vi "ParseLines.vi"(8 "error in":errorcluster, 11 "Lines":string[](array[string])) -> (0 "error out":errorcluster, 3 "Config":T1)   [LabVIEW 2020]
uses:
  <vilib>/WebServerConfig/Config.ctl
  <vilib>/WebServerConfig/Server.ctl
  <vilib>/WebServerConfig/Alias.ctl
  <vilib>/WebServerConfig/ErrorDocument.ctl
  <vilib>/WebServerConfig/Action.ctl
  <vilib>/WebServerConfig/Redirect.ctl
  <vilib>/WebServerConfig/Interface.ctl
  <vilib>/WebServerConfig/AddHandler.ctl
  <vilib>/WebServerConfig/SSL.ctl
  <vilib>/WebServerConfig/CustomLog.ctl
  <vilib>/WebServerConfig/LoadModule.ctl
  <vilib>/regexp/Match Regular Expression.xnode
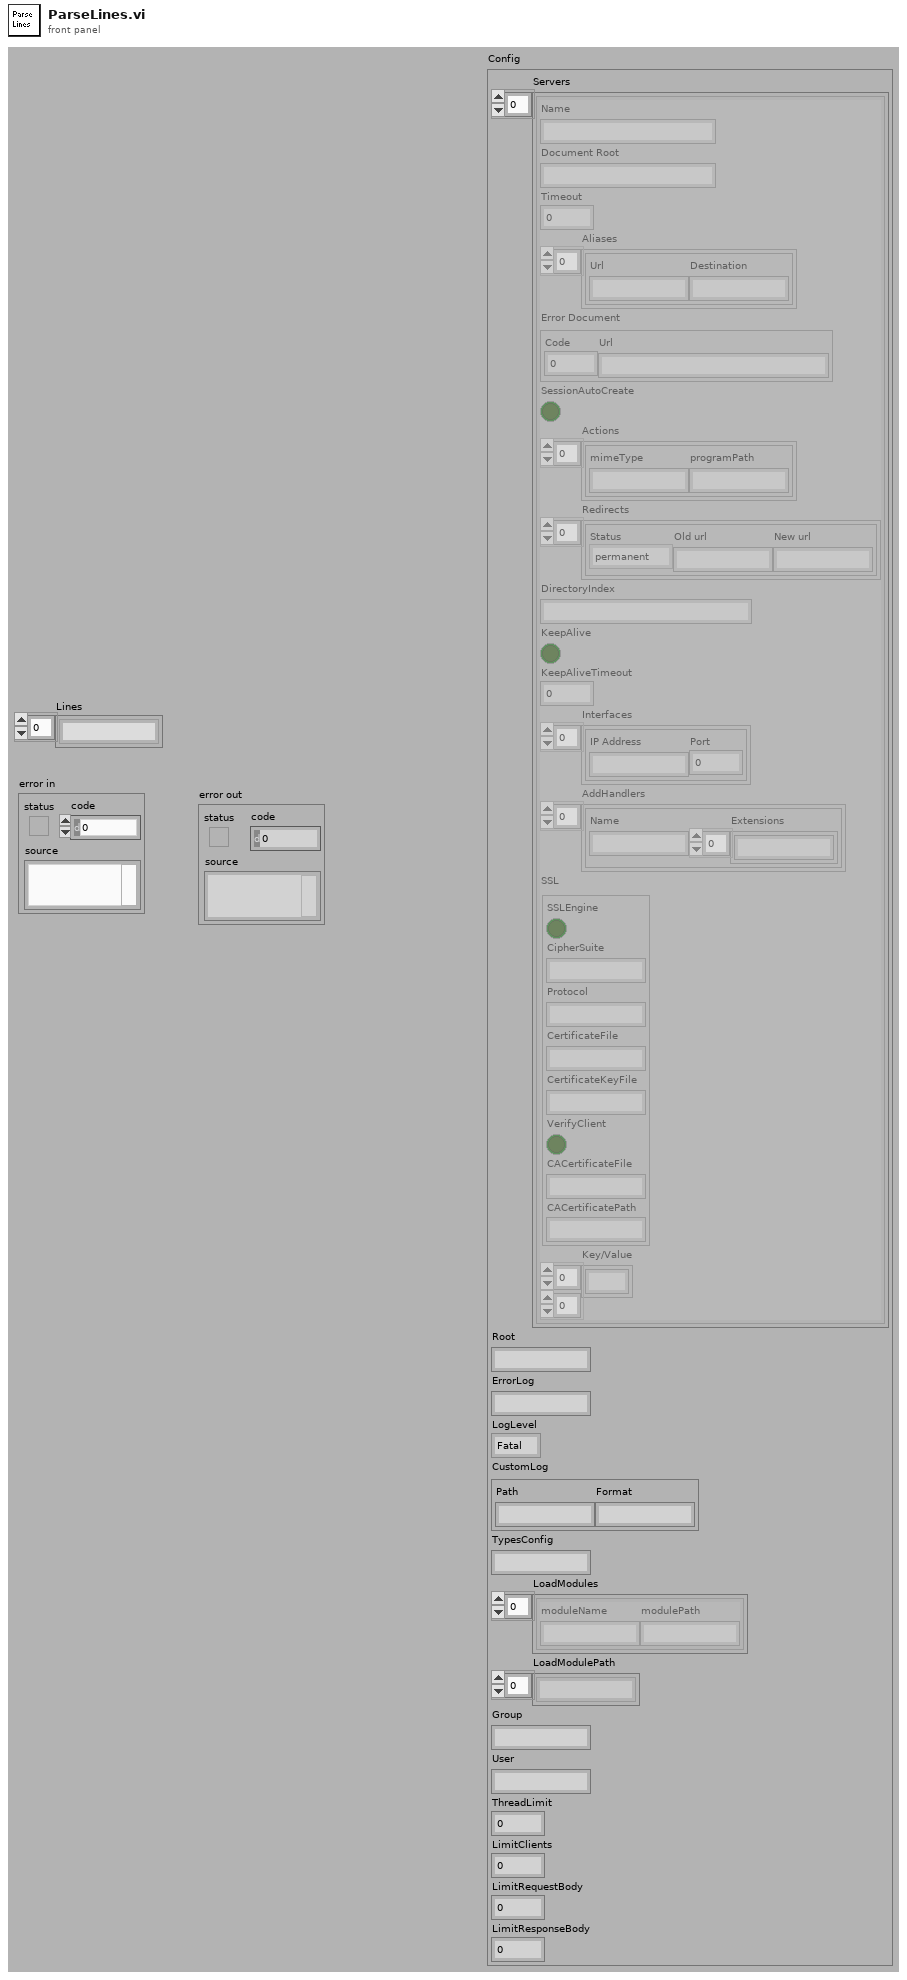
[diagram p1: front panel]
types:
  T1 = typedef "Config.ctl" = cluster{"Servers":T2[], "Root":string, "ErrorLog":string, "LogLevel":enum16{"Fatal", "Error", "Warn", "Info", "Debug", "5", "6", "7", "8", "Verbose"}, "CustomLog":T10, "TypesConfig":string, "LoadModules":T11[], "LoadModulePath":string[], "Group":string, "User":string, "ThreadLimit":u32, "LimitClients":u32, "LimitRequestBody":u32, "LimitResponseBody":u32}
  T2 = typedef "Server.ctl" = cluster{"Name":string, "Document Root":string, "Timeout":u32, "Aliases":T3[], "Error Document":T4, "SessionAutoCreate":bool, "Actions":T5[], "Redirects":T6[], "DirectoryIndex":string, "KeepAlive":bool, "KeepAliveTimeout":u32, "Interfaces":T7[], "AddHandlers":T8[], "SSL":T9, "Key/Value":string[][]}
  T3 = typedef "Alias.ctl" = cluster{"Url":string, "Destination":string}
  T4 = typedef "ErrorDocument.ctl" = cluster{"Code":u16, "Url":string}
  T5 = typedef "Action.ctl" = cluster{"mimeType":string, "programPath":string}
  T6 = typedef "Redirect.ctl" = cluster{"Status":enum16{"permanent", "temp", "seeother", "gone"}, "Old url":string, "New url":string}
  T7 = typedef "Interface.ctl" = cluster{"IP Address":string, "Port":u16}
  T8 = typedef "AddHandler.ctl" = cluster{"Name":string, "Extensions":string[]}
  T9 = typedef "SSL.ctl" = cluster{"SSLEngine":bool, "CipherSuite":string, "Protocol":string, "CertificateFile":string, "CertificateKeyFile":string, "VerifyClient":bool, "CACertificateFile":string, "CACertificatePath":string}
  T10 = typedef "CustomLog.ctl" = cluster{"Path":string, "Format":string}
  T11 = typedef "LoadModule.ctl" = cluster{"moduleName":string, "modulePath":string}
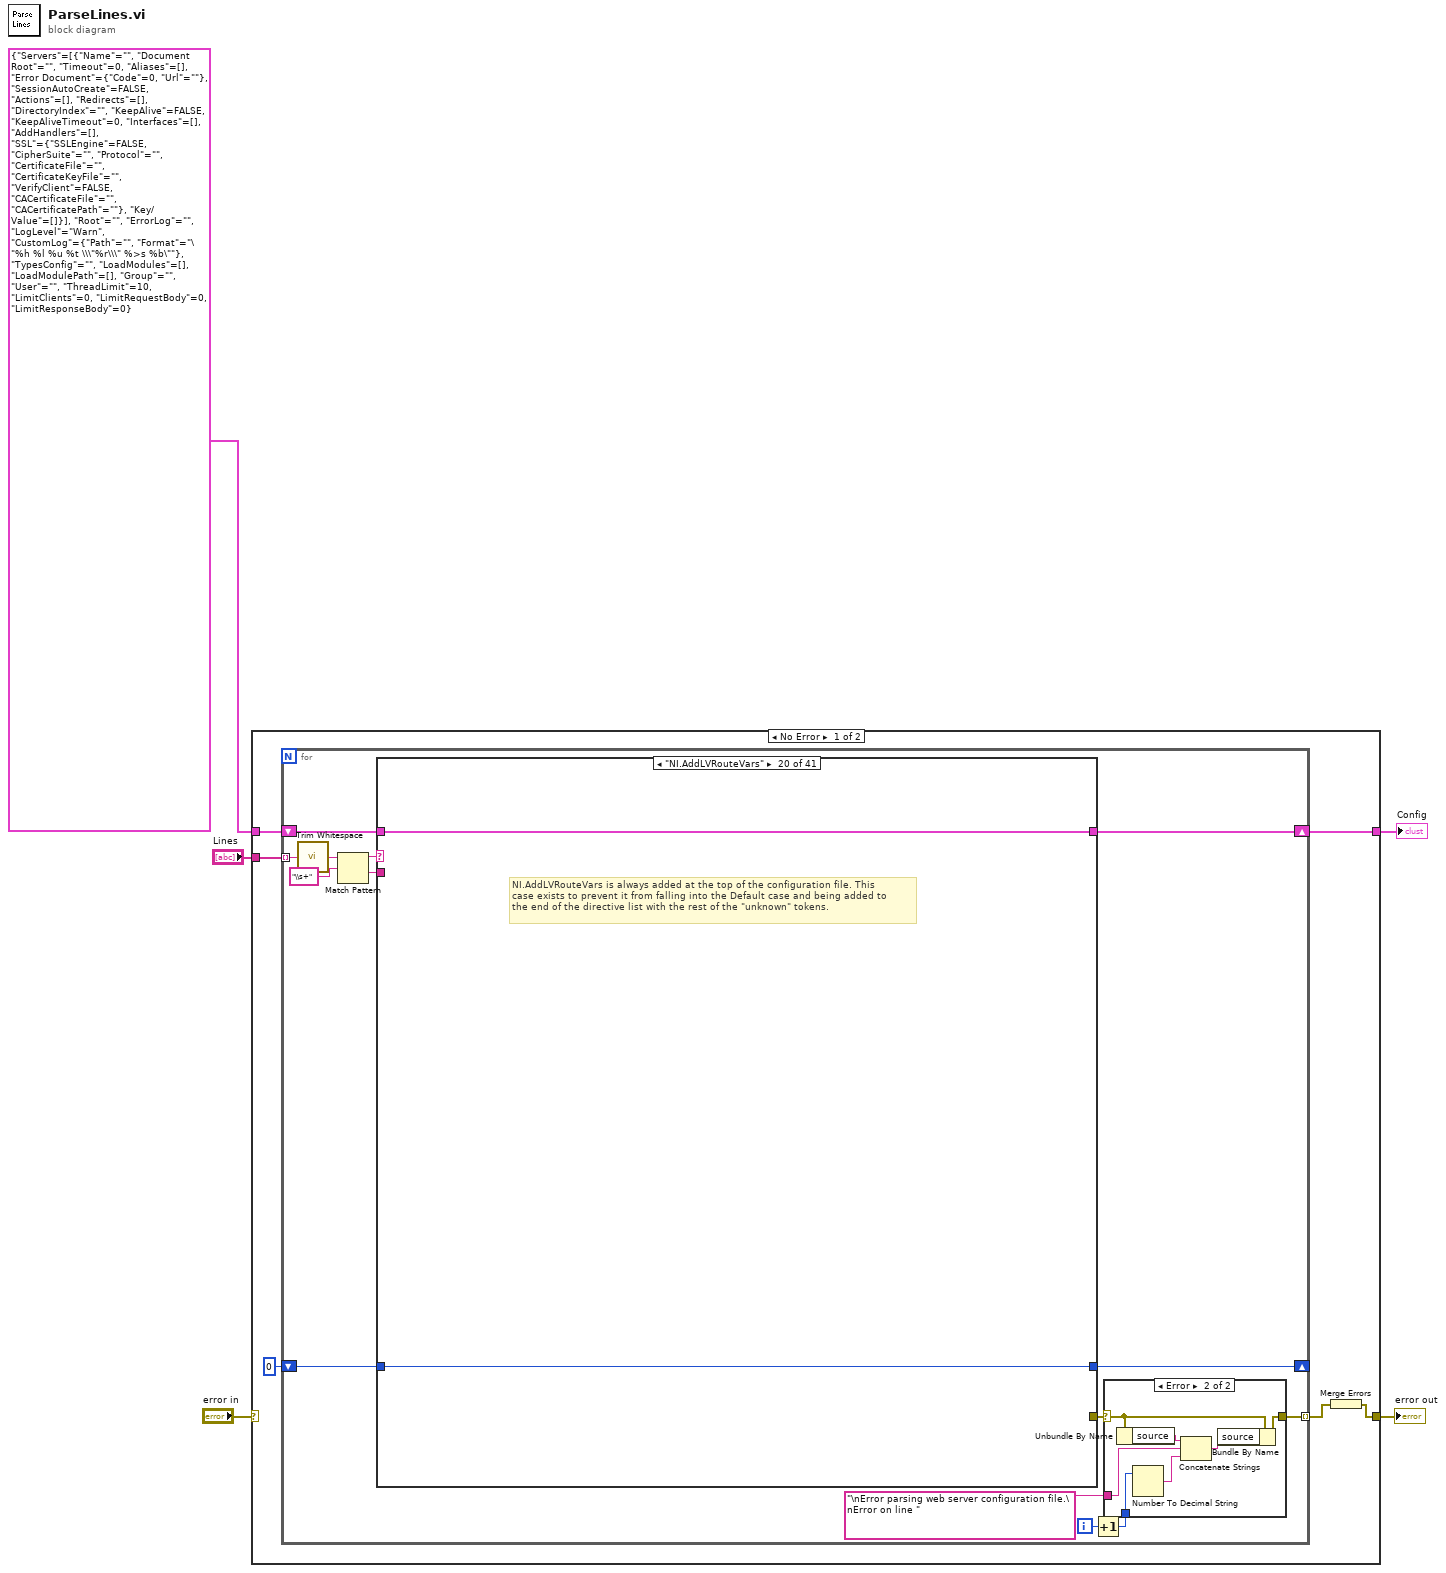
[diagram p0: block diagram]
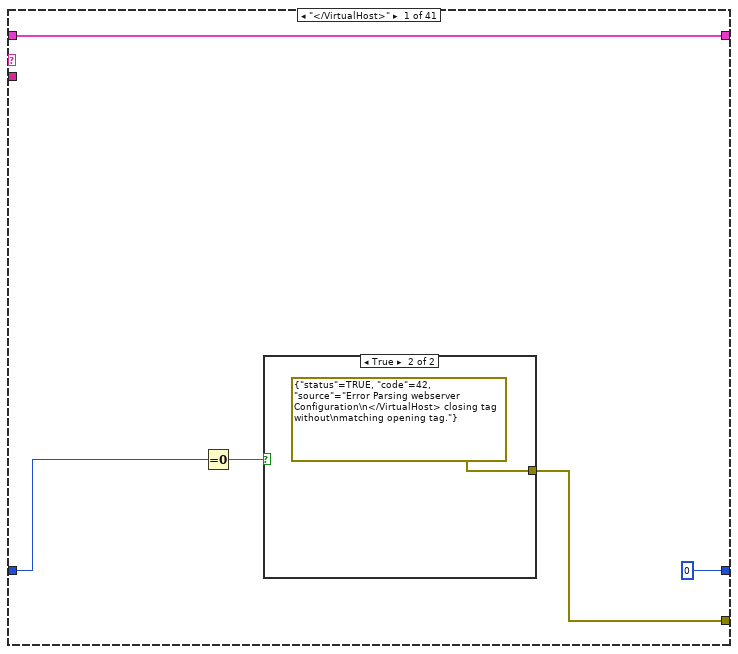
[diagram p3: hidden frame]
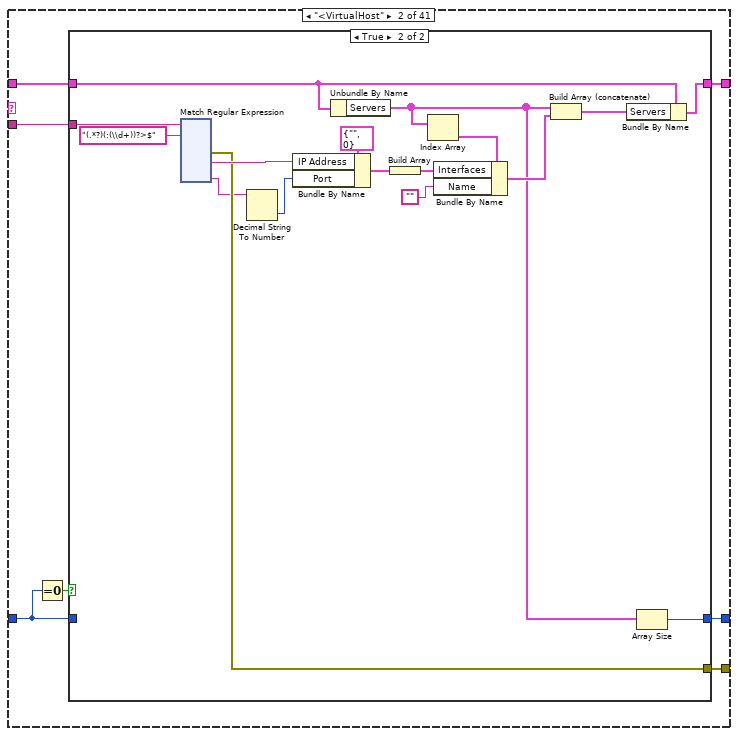
[diagram p5: hidden frame]
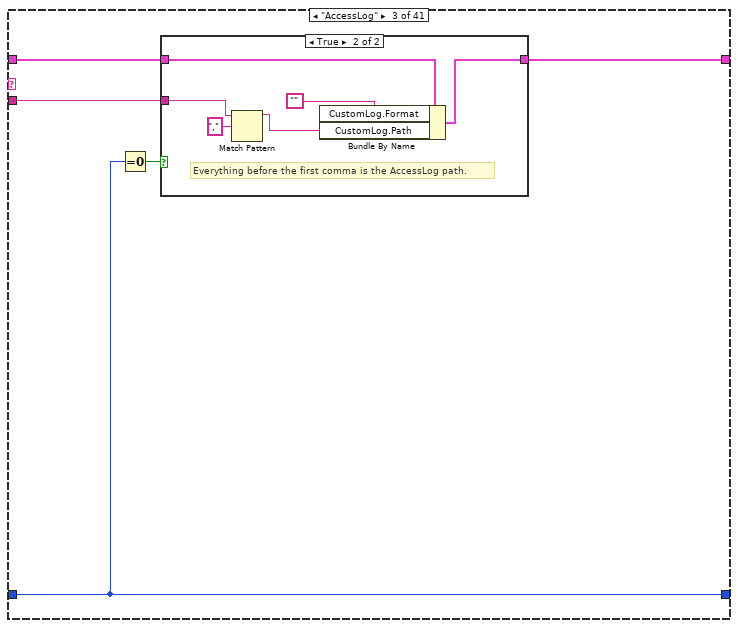
[diagram p7: hidden frame]
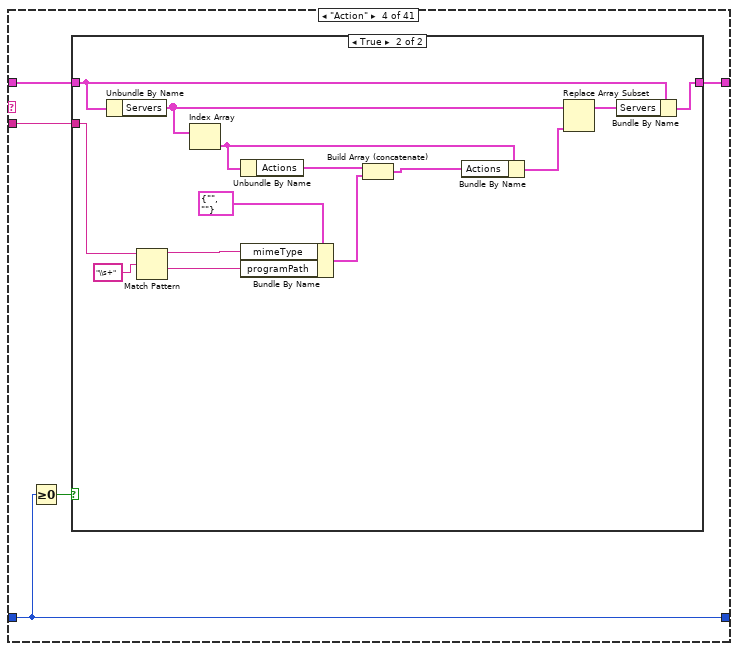
[diagram p9: hidden frame]
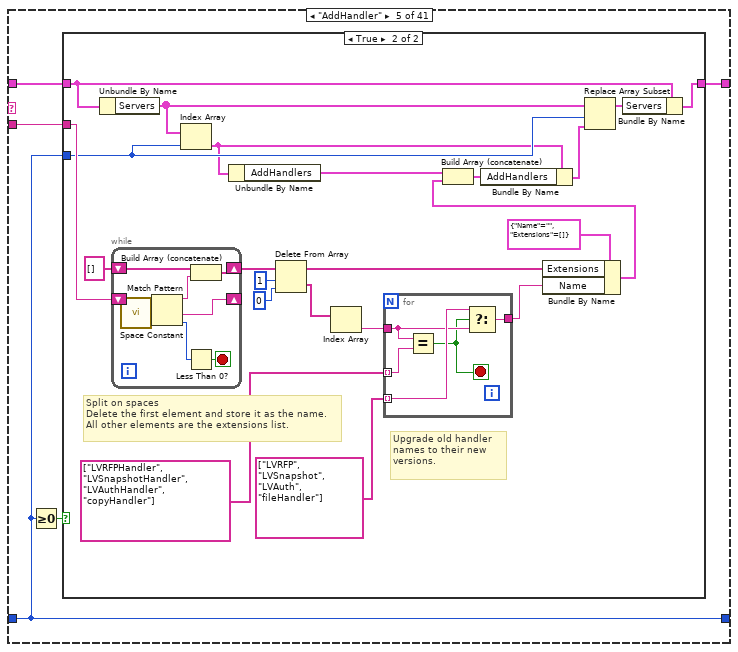
[diagram p11: hidden frame]
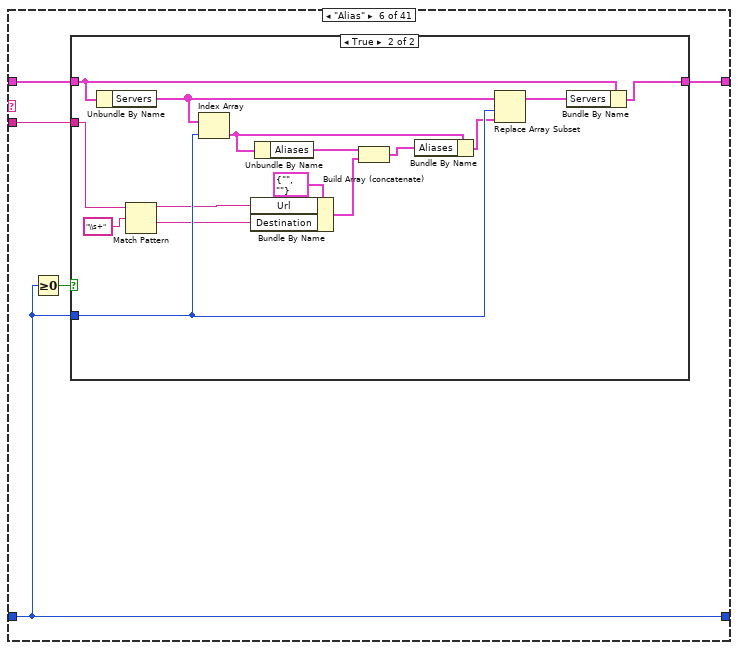
[diagram p13: hidden frame]
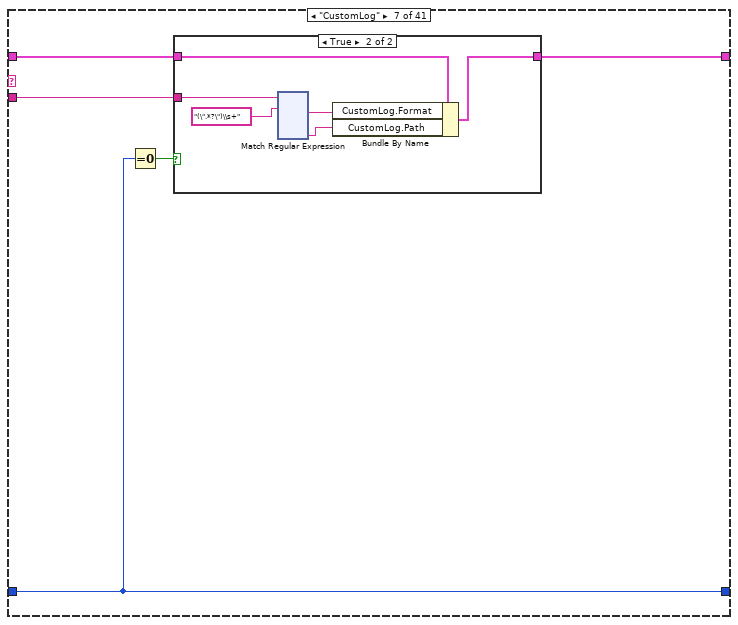
[diagram p15: hidden frame]
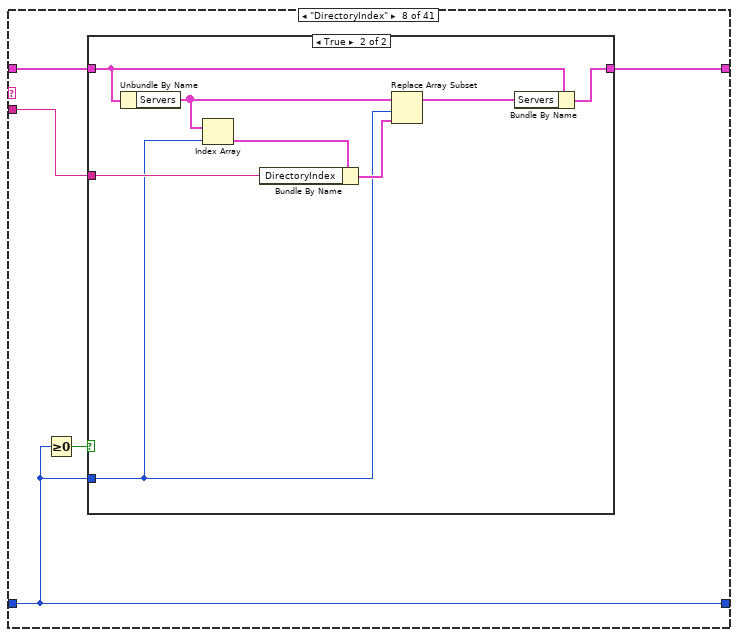
[diagram p17: hidden frame]
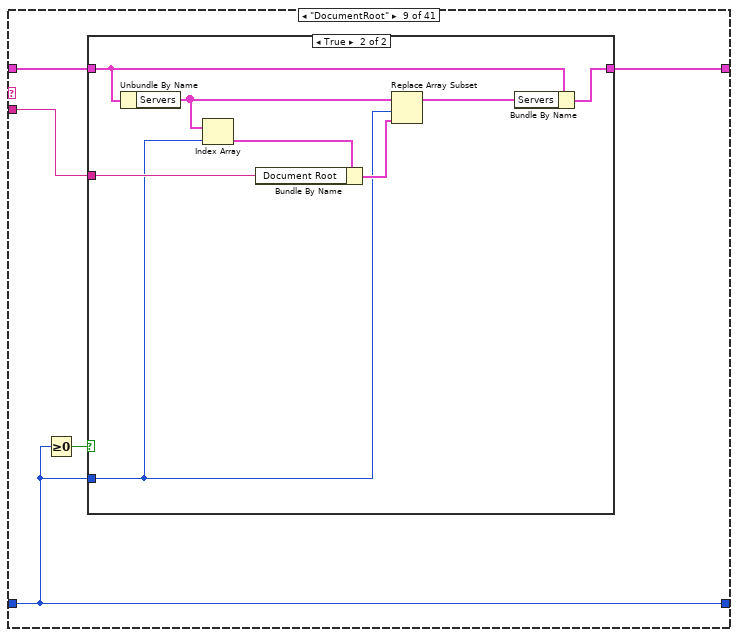
[diagram p19: hidden frame]
diagram:
  n1 = case shown="No Error" "error in" {
    selector: "error in" -> [_ w1152]
    tunnel: [w11 w1151] -> w5
    tunnel: T1 {"Servers"=[{"Name"="", "Document Root"="", "Timeout"=0, "Aliases"=[], "Error Document"={"Code"=0, "Url"=""}, "SessionAutoCreate"=FALSE, "Actions"=[], "Redirects"=[], "DirectoryIndex"="", "KeepAlive"=FALSE, "KeepAliveTimeout"=0, "Interfaces"=[], "AddHandlers"=[], "SSL"={"SSLEngine"=FALSE, "CipherSuite"="", "Protocol"="", "CertificateFile"="", "CertificateKeyFile"="", "VerifyClient"=FALSE, "CACertificateFile"="", "CACertificatePath"=""}, "Key/Value"=[]}], "Root"="", "ErrorLog"="", "LogLevel"=enum."Warn", "CustomLog"={"Path"="", "Format"="\"%h %l %u %t \\\"%r\\\" %>s %b\""}, "TypesConfig"="", "LoadModules"=[], "LoadModulePath"=[], "Group"="", "User"="", "ThreadLimit"=10, "LimitClients"=0, "LimitRequestBody"=0, "LimitResponseBody"=0} ("Config 2") -> [w9 w1151]
    tunnel: "Lines" -> [w8 _]
    tunnel: [w6 w1152] -> w2
    frame No Error {
      n2 = for {
        tunnel: w8 -> [w25] mode=indexing
        shift-right: [w20] -> w11
        shift-left: w9 -> [w21]
        shift-right: [w18] -> _
        shift-left: 0 ("CurrentServer") -> [w19]
        tunnel: [w16] -> w7 mode=indexing
        i -> [w14]
        n3 = call <vilib>:"Trim Whitespace.vi"("string"=w25) -> ("trimmed string"=w24:string)  [unwired: 1 in]
        n4 = Match Pattern(string=w24, regular expression="\\s+") -> (before substring=w22:string, after substring=w17:string)  [unwired: 1 in, 2 out]
        n5 = case shown="\"NI.AddLVRouteVars\"" w22 {
          selector: w22 -> [_ _ _ _ _ _ _ _ _ _ _ _ _ _ _ _ _ _ _ _ _ _ _ _ _ _ _ _ _ _ _ _ _ _ _ _ _ _ _ _ w1128]
          tunnel: w21 -> [w37 w45 w183 w194 w216 w256 w279 w404 w418 w430 w451 w475 w484 w500 w515 w537 w659 w689 w825 w831 w836 w864 w877 w893 w907 w921 w935 w949 w962 w977 w995 w1041 w1050 w1066 w1076 w1086 w1096 w1111 w1120 w1126 w1135]
          tunnel: [w37 w44 w182 w195 w215 w254 w278 w403 w417 w428 w449 w473 w483 w499 w514 w536 w661 w688 w823 w831 w834 w863 w875 w891 w905 w919 w933 w947 w960 w975 w992 w1039 w1049 w1065 w1075 w1085 w1095 w1109 w1118 w1126 w1134] -> w20
          tunnel: w19 -> [w35 w40 w184 w196 w213 w255 w275 w400 w414 w429 w448 w471 w480 w496 w511 w538 w658 w684 w821 w832 w835 w862 w876 w892 w906 w920 w934 w948 w961 w976 w991 w1037 w1046 w1062 w1072 w1082 w1092 w1107 w1116 w1125 w1133]
          tunnel: [0 ("CurrentServer") w43 w184 w196 w213 w255 w275 w400 w414 w429 w448 w471 w480 w496 w511 w538 w658 w684 w821 w832 w835 w862 w876 w892 w906 w920 w934 w948 w961 w976 w993 w1037 w1046 w1062 w1072 w1082 w1092 w1107 w1116 w1125 w1133] -> w18
          tunnel: w17 -> [_ w46 w181 w193 w214 w258 w277 w402 w416 w433 w450 w474 w482 w498 w513 w541 w660 w687 w824 _ w838 _ w879 w895 w909 w923 w937 _ w964 w979 w994 w1040 w1048 w1064 w1074 w1084 w1094 w1110 w1119 _ w1136]
          tunnel: [w36 w42 _ _ _ _ _ _ _ w431 _ _ _ _ _ w539 _ w686 _ _ w833 _ _ _ _ _ _ _ _ _ _ _ _ _ _ _ _ _ _ _ _] -> w13
          frame "</VirtualHost>" {
            n6 = Equal To 0?(x=w35) -> (x = 0?=w34:bool)
            n7 = case shown="True" w34 {
              tunnel: [_ errorcluster {"status"=TRUE, "code"=42, "source"="Error Parsing webserver Configuration\n</VirtualHost> closing tag without\nmatching opening tag."} ("error out")] -> w36
              frame False {
              }
              frame True {
              }
            }
          }
          frame "<VirtualHost" {
            n8 = Equal To 0?(x=w40) -> (x = 0?=w41:bool)
            n9 = case shown="True" w41 {
              tunnel: w46 -> [_ w64]
              tunnel: w45 -> [w47 w58]
              tunnel: [w47 w57] -> w44
              tunnel: [w48 w54] -> w43
              tunnel: [_ w53] -> w42
              tunnel: w40 -> [w48 _]
              frame False {
              }
              frame True {
                n10 = xnode "Match Regular Expression"("input string"=w64, "regular expression"="(.*?)(:(\\d+))?>$") -> ("error out"=w53:errorcluster, "submatch 1"=w60:string, "submatch 3"=w49:string)  [unwired: 4 in, 5 out]
                n11 = Decimal String To Number(string=w49) -> (number=w59:i32)  [unwired: 2 in, 1 out]
                n12 = Bundle By Name(cluster=T7 {"IP Address"="", "Port"=0} ("Interface"), "IP Address"=w60, "Port"=w59) -> (w62:T7)
                n13 = Unbundle By Name(w58) -> ("Servers"=w52:T2[])
                n14 = Build Array(w62) -> (w61:T7[])
                n15 = Index Array(array=w52) -> (element=w51:T2)  [unwired: 1 in]
                n16 = Bundle By Name(cluster=w51, "Interfaces"=w61, "Name"="") -> (w56:T2)
                n17 = Build Array (concatenate)(w52, w56) -> (w55:T2[])
                n18 = Bundle By Name(cluster=w58, "Servers"=w55) -> (w57:T1)
                n19 = Array Size(array=w52) -> (size(s)=w54:i32)
              }
            }
          }
          frame "AccessLog" {
            n20 = Equal To 0?(x=w184) -> (x = 0?=w185:bool)
            n21 = case shown="True" w185 {
              tunnel: [w186 w192] -> w182
              tunnel: w183 -> [w186 w191]
              tunnel: w181 -> [_ w188]
              frame False {
              }
              frame True {
                # "Everything before the first comma is the AccessLog path."
                n22 = Match Pattern(string=w188, regular expression=",") -> (before substring=w187:string)  [unwired: 1 in, 3 out]
                n23 = Bundle By Name(cluster=w191, "CustomLog.Format"="", "CustomLog.Path"=w187) -> (w192:T1)
              }
            }
          }
          frame "Action" {
            n24 = Greater Or Equal To 0?(x=w196) -> (x >= 0?=w197:bool)
            n25 = case shown="True" w197 {
              tunnel: [w198 w209] -> w195
              tunnel: w194 -> [w198 w210]
              tunnel: w193 -> [_ w211]
              frame False {
              }
              frame True {
                n26 = Unbundle By Name(w210) -> ("Servers"=w205:T2[])
                n27 = Match Pattern(string=w211, regular expression="\\s+") -> (before substring=w201:string, after substring=w200:string)  [unwired: 1 in, 2 out]
                n28 = Index Array(array=w205) -> (element=w208:T2)  [unwired: 1 in]
                n29 = Unbundle By Name(w208) -> ("Actions"=w204:T5[])
                n30 = Bundle By Name(cluster=T5 {"mimeType"="", "programPath"=""} ("Action"), "mimeType"=w201, "programPath"=w200) -> (w199:T5)
                n31 = Build Array (concatenate)(w204, w199) -> (w203:T5[])
                n32 = Bundle By Name(cluster=w208, "Actions"=w203) -> (w207:T2)
                n33 = Replace Array Subset(array=w205, new element=w207) -> (w206:T2[])  [unwired: 1 in]
                n34 = Bundle By Name(cluster=w210, "Servers"=w206) -> (w209:T1)
              }
            }
          }
          frame "AddHandler" {
            n35 = Greater Or Equal To 0?(x=w213) -> (x >= 0?=w217:bool)
            n36 = case shown="True" w217 {
              tunnel: w216 -> [w218 w235]
              tunnel: [w218 w234] -> w215
              tunnel: w214 -> [_ w240]
              tunnel: w213 -> [_ w231]
              frame False {
              }
              frame True {
                # "Upgrade old handler names to their new versions."
                # "Split on spaces\nDelete the first element and store it as the name.\nAll other elements are the extensions list."
                n37 = Unbundle By Name(w235) -> ("Servers"=w233:T2[])
                n38 = while {
                  shift-right: [w251] -> _
                  shift-left: w240 -> [w253]
                  shift-right: [w247] -> w238
                  shift-left: string[] [] -> [w246]
                  stop <- w250 stop-if-true
                  n39 = call <vilib>:"Space Constant.vi"() -> ("String"=w252:string)
                  n40 = Match Pattern(string=w253, regular expression=w252) -> (before substring=w248:string, after substring=w251:string, offset past match=w249:i32)  [unwired: 1 in, 1 out]
                  n41 = Less Than 0?(x=w249) -> (x < 0?=w250:bool)
                  n42 = Build Array (concatenate)(w246, w248) -> (w247:string[])
                }
                n43 = Index Array(array=w233, index=w231) -> (element=w230:T2)
                n44 = Unbundle By Name(w230) -> ("AddHandlers"=w228:T8[])
                n45 = Delete From Array(array=w238, length=1, index=0) -> (deleted portion=w223:string[], array with subset deleted=w224:string[])
                n46 = Index Array(array=w223) -> (element=w220:string)  [unwired: 1 in]
                n47 = for {
                  tunnel: string[] ["LVRFPHandler", "LVSnapshotHandler", "LVAuthHandler", "copyHandler"] -> [w245] mode=indexing
                  tunnel: string[] ["LVRFP", "LVSnapshot", "LVAuth", "fileHandler"] -> [w244] mode=indexing
                  tunnel: w220 -> [w243]
                  tunnel: [w242] -> w219
                  stop <- w241 stop-if-true
                  n48 = Equal?(x=w243, y=w245) -> (x = y?=w241:bool)
                  n49 = Select(t=w244, s=w241, f=w243) -> (s? t:f=w242:string)
                }
                n50 = Bundle By Name(cluster=T8 {"Name"="", "Extensions"=[]} ("AddHandler"), "Extensions"=w224, "Name"=w219) -> (w225:T8)
                n51 = Build Array (concatenate)(w228, w225) -> (w227:T8[])
                n52 = Bundle By Name(cluster=w230, "AddHandlers"=w227) -> (w229:T2)
                n53 = Replace Array Subset(array=w233, new element=w229, index=w231) -> (w232:T2[])
                n54 = Bundle By Name(cluster=w235, "Servers"=w232) -> (w234:T1)
              }
            }
          }
          frame "Alias" {
            n55 = Greater Or Equal To 0?(x=w255) -> (x >= 0?=w257:bool)
            n56 = case shown="True" w257 {
              tunnel: w258 -> [_ w273]
              tunnel: w256 -> [w259 w272]
              tunnel: w255 -> [_ w268]
              tunnel: [w259 w271] -> w254
              frame False {
              }
              frame True {
                n57 = Unbundle By Name(w272) -> ("Servers"=w269:T2[])
                n58 = Match Pattern(string=w273, regular expression="\\s+") -> (before substring=w266:string, after substring=w265:string)  [unwired: 1 in, 2 out]
                n59 = Index Array(array=w269, index=w268) -> (element=w264:T2)
                n60 = Bundle By Name(cluster=T3 {"Url"="", "Destination"=""} ("Alias"), "Url"=w266, "Destination"=w265) -> (w260:T3)
                n61 = Unbundle By Name(w264) -> ("Aliases"=w262:T3[])
                n62 = Build Array (concatenate)(w262, w260) -> (w261:T3[])
                n63 = Bundle By Name(cluster=w264, "Aliases"=w261) -> (w263:T2)
                n64 = Replace Array Subset(array=w269, new element=w263, index=w268) -> (w270:T2[])
                n65 = Bundle By Name(cluster=w272, "Servers"=w270) -> (w271:T1)
              }
            }
          }
          frame "CustomLog" {
            n66 = Equal To 0?(x=w275) -> (x = 0?=w276:bool)
            n67 = case shown="True" w276 {
              tunnel: w279 -> [w280 w286]
              tunnel: [w280 w285] -> w278
              tunnel: w277 -> [_ w283]
              frame False {
              }
              frame True {
                n68 = xnode "Match Regular Expression"("input string"=w283, "regular expression"="(\".*?\")\\s+") -> ("after match"=w282:string, "submatch 1"=w281:string)  [unwired: 4 in, 4 out]
                n69 = Bundle By Name(cluster=w286, "CustomLog.Format"=w282, "CustomLog.Path"=w281) -> (w285:T1)
              }
            }
          }
          frame "DirectoryIndex" {
            n70 = Greater Or Equal To 0?(x=w400) -> (x >= 0?=w401:bool)
            n71 = case shown="True" w401 {
              tunnel: w404 -> [w405 w413]
              tunnel: [w405 w411] -> w403
              tunnel: w402 -> [_ w409]
              tunnel: w400 -> [_ w406]
              frame False {
              }
              frame True {
                n72 = Unbundle By Name(w413) -> ("Servers"=w407:T2[])
                n73 = Index Array(array=w407, index=w406) -> (element=w410:T2)
                n74 = Bundle By Name(cluster=w410, "DirectoryIndex"=w409) -> (w408:T2)
                n75 = Replace Array Subset(array=w407, new element=w408, index=w406) -> (w412:T2[])
                n76 = Bundle By Name(cluster=w413, "Servers"=w412) -> (w411:T1)
              }
            }
          }
          frame "DocumentRoot" {
            n77 = Greater Or Equal To 0?(x=w414) -> (x >= 0?=w415:bool)
            n78 = case shown="True" w415 {
              tunnel: w418 -> [w419 w427]
              tunnel: [w419 w425] -> w417
              tunnel: w416 -> [_ w423]
              tunnel: w414 -> [_ w420]
              frame False {
              }
              frame True {
                n79 = Unbundle By Name(w427) -> ("Servers"=w421:T2[])
                n80 = Index Array(array=w421, index=w420) -> (element=w424:T2)
                n81 = Bundle By Name(cluster=w424, "Document Root"=w423) -> (w422:T2)
                n82 = Replace Array Subset(array=w421, new element=w422, index=w420) -> (w426:T2[])
                n83 = Bundle By Name(cluster=w427, "Servers"=w426) -> (w425:T1)
              }
            }
          }
          frame "ErrorDocument" {
            n84 = Greater Or Equal To 0?(x=w429) -> (x >= 0?=w432:bool)
            n85 = case shown="True" w432 {
              tunnel: w433 -> [_ w446]
              tunnel: [_ w444] -> w431
              tunnel: w430 -> [w434 w443]
              tunnel: w429 -> [_ w440]
              tunnel: [w434 w442] -> w428
              frame False {
              }
              frame True {
                n86 = Unbundle By Name(w443) -> ("Servers"=w441:T2[])
                n87 = Scan From String(format string="%d %s", input string=w446) -> (error out=w444:errorcluster, output 1=w437:i32, output 2=w436:string)  [unwired: 4 in, 2 out]
                n88 = Index Array(array=w441, index=w440) -> (element=w438:T2)
                n89 = Bundle By Name(cluster=w438, "Error Document.Code"=w437, "Error Document.Url"=w436) -> (w435:T2)
                n90 = Replace Array Subset(array=w441, new element=w435, index=w440) -> (w439:T2[])
                n91 = Bundle By Name(cluster=w443, "Servers"=w439) -> (w442:T1)
              }
            }
          }
          frame "ErrorLog" {
            n92 = Equal To 0?(x=w448) -> (x = 0?=w447:bool)
            n93 = case shown="True" w447 {
              tunnel: w451 -> [w452 w463]
              tunnel: w450 -> [_ w461]
              tunnel: [w452 w453] -> w449
              frame False {
              }
              frame True {
                # "Everything before the first comma is the log path. If the logspec contains a level\ndeclaration, use that as the LogLevel."
                n94 = Match Pattern(string=w461, regular expression=",") -> (before substring=w460:string, after substring=w459:string)  [unwired: 1 in, 2 out]
                n95 = Bundle By Name(cluster=w463, "ErrorLog"=w460) -> (w454:T1)
                n96 = Match Pattern(string=w459, regular expression="level=") -> (after substring=w457:string, offset past match=w456:i32)  [unwired: 1 in, 2 out]
                n97 = Greater Or Equal To 0?(x=w456) -> (x >= 0?=w455:bool)
                n98 = case shown="True" w455 {
                  tunnel: w457 -> [_ w469]
                  tunnel: w454 -> [w464 w468]
                  tunnel: [w464 w467] -> w453
                  frame False {
                  }
                  frame True {
                    n99 = Match Pattern(string=w469, regular expression=",") -> (before substring=w466:string)  [unwired: 1 in, 3 out]
                    n100 = Decimal String To Number(string=w466) -> (number=w465:i32)  [unwired: 2 in, 1 out]
                    n101 = Bundle By Name(cluster=w468, "LogLevel"=w465) -> (w467:T1)
                  }
                }
              }
            }
          }
          frame "Group" {
            n102 = Equal To 0?(x=w471) -> (x = 0?=w472:bool)
            n103 = case shown="True" w472 {
              tunnel: w475 -> [w476 w479]
              tunnel: w474 -> [_ w478]
              tunnel: [w476 w477] -> w473
              frame False {
              }
              frame True {
                n104 = Bundle By Name(cluster=w479, "Group"=w478) -> (w477:T1)
              }
            }
          }
          frame "KeepAlive" {
            n105 = Greater Or Equal To 0?(x=w480) -> (x >= 0?=w481:bool)
            n106 = case shown="True" w481 {
              tunnel: w484 -> [w485 w495]
              tunnel: [w485 w493] -> w483
              tunnel: w482 -> [_ w488]
              tunnel: w480 -> [_ w489]
              frame False {
              }
              frame True {
                n107 = Unbundle By Name(w495) -> ("Servers"=w490:T2[])
                n108 = Equal?(x=w488, y="on") -> (x = y?=w487:bool)
                n109 = Index Array(array=w490, index=w489) -> (element=w492:T2)
                n110 = Bundle By Name(cluster=w492, "KeepAlive"=w487) -> (w491:T2)
                n111 = Replace Array Subset(array=w490, new element=w491, index=w489) -> (w494:T2[])
                n112 = Bundle By Name(cluster=w495, "Servers"=w494) -> (w493:T1)
              }
            }
          }
          frame "KeepAliveTimeout" {
            n113 = Greater Or Equal To 0?(x=w496) -> (x >= 0?=w497:bool)
            n114 = case shown="True" w497 {
              tunnel: w500 -> [w501 w510]
              tunnel: [w501 w508] -> w499
              tunnel: w498 -> [_ w503]
              tunnel: w496 -> [_ w504]
              frame False {
              }
              frame True {
                n115 = Unbundle By Name(w510) -> ("Servers"=w505:T2[])
                n116 = Decimal String To Number(string=w503) -> (number=w502:i32)  [unwired: 2 in, 1 out]
                n117 = Index Array(array=w505, index=w504) -> (element=w507:T2)
                n118 = Bundle By Name(cluster=w507, "KeepAliveTimeout"=w502) -> (w506:T2)
                n119 = Replace Array Subset(array=w505, new element=w506, index=w504) -> (w509:T2[])
                n120 = Bundle By Name(cluster=w510, "Servers"=w509) -> (w508:T1)
              }
            }
          }
          frame "LimitClients" {
            n121 = Equal To 0?(x=w511) -> (x = 0?=w512:bool)
            n122 = case shown="True" w512 {
              tunnel: w515 -> [w516 w520]
              tunnel: [w516 w519] -> w514
              tunnel: w513 -> [_ w518]
              frame False {
              }
              frame True {
                n123 = Decimal String To Number(string=w518) -> (number=w517:i32)  [unwired: 2 in, 1 out]
                n124 = Bundle By Name(cluster=w520, "LimitClients"=w517) -> (w519:T1)
              }
            }
          }
          frame "Listen" {
            w533 = 0
            # "This one is odd.\nWe'll take it at any level"
            # "Add all listens as interfaces on the default server.\nAfter parsing all the lines the interfaces that are\nused by virtual hosts will be removed from the\ndefault server's set."
            n125 = Unbundle By Name(w537) -> ("Servers"=w535:T2[])
            n126 = xnode "Match Regular Expression"("input string"=w541, "regular expression"="((.*):)?(\\d+)") -> ("error out"=w539:errorcluster, "submatch 2"=w523:string, "submatch 3"=w526:string)  [unwired: 4 in, 5 out]
            n127 = Decimal String To Number(string=w526) -> (number=w525:i32)  [unwired: 2 in, 1 out]
            n128 = Empty String/Path?(string/path=w523) -> (empty?=w524:bool)
            n129 = Index Array(array=w535, index=w533) -> (element=w531:T2)
            n130 = Select(t="*", s=w524, f=w523) -> (s? t:f=w522:string)
            n131 = Unbundle By Name(w531) -> ("Interfaces"=w530:T7[])
            n132 = Bundle By Name(cluster=T7 {"IP Address"="", "Port"=0} ("Interface"), "IP Address"=w522, "Port"=w525) -> (w527:T7)
            n133 = Build Array (concatenate)(w530, w527) -> (w529:T7[])
            n134 = Bundle By Name(cluster=w531, "Interfaces"=w529) -> (w532:T2)
            n135 = Replace Array Subset(array=w535, new element=w532, index=w533) -> (w534:T2[])
            n136 = Bundle By Name(cluster=w537, "Servers"=w534) -> (w536:T1)
          }
          frame "LoadModule" {
            n137 = Equal To 0?(x=w658) -> (x = 0?=w657:bool)
            n138 = case shown="True" w657 {
              tunnel: [w662 w670] -> w661
              tunnel: w660 -> [_ w668]
              tunnel: w659 -> [w662 w667]
              frame False {
              }
              frame True {
                n139 = Match Pattern(string=w668, regular expression="\\s+") -> (before substring=w663:string, after substring=w665:string)  [unwired: 1 in, 2 out]
                n140 = Bundle By Name(cluster=T11 {"moduleName"="", "modulePath"=""} ("LoadModule"), "moduleName"=w663, "modulePath"=w665) -> (w664:T11)
                n141 = case shown="Default" w663 {
                  tunnel: [w677 w682 w683] -> w670
                  tunnel: w667 -> [w676 w682 w683]
                  tunnel: w664 -> [w671 _ _]
                  frame Default {
                    # "Load Modules should be unique. Only add it if it isn't already in the list"
                    n142 = Unbundle By Name(w676) -> ("LoadModules"=w674:T11[])
                    n143 = Search 1D Array(1D array=w674, element=w671) -> (index of element=w672:i32)  [unwired: 1 in]
                    n144 = Less Than 0?(x=w672) -> (x < 0?=w673:bool)
                    n145 = case shown="True" w673 {
                      tunnel: [w678 w681] -> w675
                      tunnel: w674 -> [w678 w680]
                      tunnel: w671 -> [_ w679]
                      frame False {
                      }
                      frame True {
                        n146 = Build Array (concatenate)(w680, w679) -> (w681:T11[])
                      }
                    }
                    n147 = Bundle By Name(cluster=w676, "LoadModules"=w675) -> (w677:T1)
                  }
                  frame "copy" {
                    # "The \"copyModule\" is built in as of Appweb 4;\ndon't generate a LoadModule directive for it."
                  }
                  frame "dir" {
                    # "The \"dirModule\" is built in as of Appweb 4;\ndon't generate a LoadModule directive for it."
                  }
                }
              }
            }
          }
          frame "LoadModulePath" {
            n148 = Equal To 0?(x=w684) -> (x = 0?=w685:bool)
            n149 = case shown="True" w685 {
              tunnel: w689 -> [w690 w696]
              tunnel: [w690 w695] -> w688
              tunnel: w687 -> [_ w694]
              tunnel: [_ w691] -> w686
              frame False {
              }
              frame True {
                n150 = while {
                  shift-right: [w700] -> _
                  shift-left: w694 -> [w707]
                  shift-right: [w698] -> w692
                  shift-left: string[] [] -> [w699]
                  tunnel: [w705] -> w691
                  stop <- w701 stop-if-true
                  n151 = xnode "Match Regular Expression"("input string"=w707, "regular expression"="(\".*?\"|.*?)(\\s+|$)") -> ("after match"=w700:string, "offset past match"=w706:i32, "error out"=w705:errorcluster, "submatch 1"=w697:string)  [unwired: 4 in, 2 out]
                  n152 = Build Array (concatenate)(w699, w697) -> (w698:string[])
                  n153 = Empty String/Path?(string/path=w700) -> (empty?=w702:bool)
                  n154 = Less Than 0?(x=w706) -> (x < 0?=w703:bool)
                  n155 = Or(x=w702, y=w703) -> (x .or. y?=w701:bool)
                }
                n156 = Bundle By Name(cluster=w696, "LoadModulePath"=w692) -> (w695:T1)
              }
            }
          }
          frame "LogLevel" {
            n157 = Equal To 0?(x=w821) -> (x = 0?=w822:bool)
            n158 = case shown="True" w822 {
              tunnel: w825 -> [w826 w830]
              tunnel: w824 -> [_ w829]
              tunnel: [w826 w828] -> w823
              frame False {
              }
              frame True {
                n159 = Decimal String To Number(string=w829) -> (number=w827:i32)  [unwired: 2 in, 1 out]
                n160 = Bundle By Name(cluster=w830, "LogLevel"=w827) -> (w828:T1)
              }
            }
          }
          frame "NI.AddLVRouteVars" {
            # "NI.AddLVRouteVars is always added at the top of the configuration file. This\ncase exists to prevent it from falling into the Default case and being added to\nthe end of the directive list with the rest of the \"unknown\" tokens."
          }
          frame "Redirect" {
            n161 = Greater Or Equal To 0?(x=w835) -> (x >= 0?=w837:bool)
            n162 = case shown="True" w837 {
              tunnel: w838 -> [_ w846]
              tunnel: w836 -> [w839 w857]
              tunnel: w835 -> [_ w853]
              tunnel: [w839 w856] -> w834
              tunnel: [_ w842] -> w833
              frame False {
              }
              frame True {
                n163 = Unbundle By Name(w857) -> ("Servers"=w854:T2[])
                n164 = Scan From String(format string="%d %s %s", input string=w846) -> (error out=w842:errorcluster, output 1=w841:i32, output 2=w844:string, output 3=w843:string)  [unwired: 5 in, 2 out]
                n165 = case shown="301, Default" w841 {
                  tunnel: [enum16{"permanent", "temp", "seeother", "gone"}."temp" ("Status") enum16{"permanent", "temp", "seeother", "gone"}."seeother" ("Status") enum16{"permanent", "temp", "seeother", "gone"}."gone" ("Status") enum16{"permanent", "temp", "seeother", "gone"}."permanent" ("Status")] -> w840
                  frame 302 {
                  }
                  frame 303 {
                  }
                  frame 410 {
                  }
                  frame 301, Default {
                  }
                }
                n166 = Index Array(array=w854, index=w853) -> (element=w852:T2)
                n167 = Unbundle By Name(w852) -> ("Redirects"=w850:T6[])
                n168 = Bundle By Name(cluster=T6 {"Status"=enum."permanent", "Old url"="", "New url"=""} ("Redirect"), "Old url"=w844, "New url"=w843, "Status"=w840) -> (w848:T6)
                n169 = Build Array (concatenate)(w850, w848) -> (w849:T6[])
                n170 = Bundle By Name(cluster=w852, "Redirects"=w849) -> (w851:T2)
                n171 = Replace Array Subset(array=w854, new element=w851, index=w853) -> (w855:T2[])
                n172 = Bundle By Name(cluster=w857, "Servers"=w855) -> (w856:T1)
              }
            }
          }
          frame "ResetHandlers" {
            n173 = Greater Than 0?(x=w862) -> (x > 0?=w865:bool)
            n174 = case shown="True" w865 {
              tunnel: w864 -> [w866 w874]
              tunnel: [w866 w873] -> w863
              tunnel: w862 -> [_ w870]
              frame False {
              }
              frame True {
                n175 = Unbundle By Name(w874) -> ("Servers"=w872:T2[])
                n176 = Index Array(array=w872, index=w870) -> (element=w869:T2)
                n177 = Bundle By Name(cluster=w869, "AddHandlers"=T8[] []) -> (w868:T2)
                n178 = Replace Array Subset(array=w872, new element=w868, index=w870) -> (w871:T2[])
                n179 = Bundle By Name(cluster=w874, "Servers"=w871) -> (w873:T1)
              }
            }
          }
          frame "SSLEngine" {
            n180 = Greater Or Equal To 0?(x=w876) -> (x >= 0?=w878:bool)
            n181 = case shown="True" w878 {
              tunnel: w879 -> [_ w883]
              tunnel: w877 -> [w880 w890]
              tunnel: w876 -> [_ w886]
              tunnel: [w880 w889] -> w875
              frame False {
              }
              frame True {
                n182 = Unbundle By Name(w890) -> ("Servers"=w887:T2[])
                n183 = Index Array(array=w887, index=w886) -> (element=w885:T2)
                n184 = Equal?(x=w883, y="on") -> (x = y?=w882:bool)
                n185 = Bundle By Name(cluster=w885, "SSL.SSLEngine"=w882) -> (w884:T2)
                n186 = Replace Array Subset(array=w887, new element=w884, index=w886) -> (w888:T2[])
                n187 = Bundle By Name(cluster=w890, "Servers"=w888) -> (w889:T1)
              }
            }
          }
          frame "SSLCipherSuite" {
            n188 = Greater Or Equal To 0?(x=w892) -> (x >= 0?=w894:bool)
            n189 = case shown="True" w894 {
              tunnel: w895 -> [_ w897]
              tunnel: w893 -> [w896 w904]
              tunnel: w892 -> [_ w900]
              tunnel: [w896 w903] -> w891
              frame False {
              }
              frame True {
                n190 = Unbundle By Name(w904) -> ("Servers"=w901:T2[])
                n191 = Index Array(array=w901, index=w900) -> (element=w899:T2)
                n192 = Bundle By Name(cluster=w899, "SSL.CipherSuite"=w897) -> (w898:T2)
                n193 = Replace Array Subset(array=w901, new element=w898, index=w900) -> (w902:T2[])
                n194 = Bundle By Name(cluster=w904, "Servers"=w902) -> (w903:T1)
              }
            }
          }
          frame "SSLProtocol" {
            n195 = Greater Or Equal To 0?(x=w906) -> (x >= 0?=w908:bool)
            n196 = case shown="True" w908 {
              tunnel: w909 -> [_ w911]
              tunnel: w907 -> [w910 w918]
              tunnel: w906 -> [_ w914]
              tunnel: [w910 w917] -> w905
              frame False {
              }
              frame True {
                n197 = Unbundle By Name(w918) -> ("Servers"=w915:T2[])
                n198 = Index Array(array=w915, index=w914) -> (element=w913:T2)
                n199 = Bundle By Name(cluster=w913, "SSL.Protocol"=w911) -> (w912:T2)
                n200 = Replace Array Subset(array=w915, new element=w912, index=w914) -> (w916:T2[])
                n201 = Bundle By Name(cluster=w918, "Servers"=w916) -> (w917:T1)
              }
            }
          }
          frame "SSLCertificateFile" {
            n202 = Greater Or Equal To 0?(x=w920) -> (x >= 0?=w922:bool)
            n203 = case shown="True" w922 {
              tunnel: w923 -> [_ w925]
              tunnel: w921 -> [w924 w932]
              tunnel: w920 -> [_ w928]
              tunnel: [w924 w931] -> w919
              frame False {
              }
              frame True {
                n204 = Unbundle By Name(w932) -> ("Servers"=w929:T2[])
                n205 = Index Array(array=w929, index=w928) -> (element=w927:T2)
                n206 = Bundle By Name(cluster=w927, "SSL.CertificateFile"=w925) -> (w926:T2)
                n207 = Replace Array Subset(array=w929, new element=w926, index=w928) -> (w930:T2[])
                n208 = Bundle By Name(cluster=w932, "Servers"=w930) -> (w931:T1)
              }
            }
          }
          frame "SSLCertificateKeyFile" {
            n209 = Greater Or Equal To 0?(x=w934) -> (x >= 0?=w936:bool)
            n210 = case shown="True" w936 {
              tunnel: w937 -> [_ w939]
              tunnel: w935 -> [w938 w946]
              tunnel: w934 -> [_ w942]
              tunnel: [w938 w945] -> w933
              frame False {
              }
              frame True {
                n211 = Unbundle By Name(w946) -> ("Servers"=w943:T2[])
                n212 = Index Array(array=w943, index=w942) -> (element=w941:T2)
                n213 = Bundle By Name(cluster=w941, "SSL.CertificateKeyFile"=w939) -> (w940:T2)
                n214 = Replace Array Subset(array=w943, new element=w940, index=w942) -> (w944:T2[])
                n215 = Bundle By Name(cluster=w946, "Servers"=w944) -> (w945:T1)
              }
            }
          }
          frame "SSLVerifyClient" {
            n216 = Greater Or Equal To 0?(x=w948) -> (x >= 0?=w950:bool)
            n217 = case shown="True" w950 {
              tunnel: w949 -> [w951 w959]
              tunnel: w948 -> [_ w955]
              tunnel: [w951 w958] -> w947
              frame False {
              }
              frame True {
                n218 = Unbundle By Name(w959) -> ("Servers"=w956:T2[])
                n219 = Index Array(array=w956, index=w955) -> (element=w954:T2)
                n220 = Bundle By Name(cluster=w954, "SSL.VerifyClient"=TRUE) -> (w953:T2)
                n221 = Replace Array Subset(array=w956, new element=w953, index=w955) -> (w957:T2[])
                n222 = Bundle By Name(cluster=w959, "Servers"=w957) -> (w958:T1)
              }
            }
          }
          frame "SSLCACertificateFile" {
            n223 = Greater Or Equal To 0?(x=w961) -> (x >= 0?=w963:bool)
            n224 = case shown="True" w963 {
              tunnel: w964 -> [_ w967]
              tunnel: w962 -> [w965 w974]
              tunnel: w961 -> [_ w970]
              tunnel: [w965 w973] -> w960
              frame False {
              }
              frame True {
                n225 = Unbundle By Name(w974) -> ("Servers"=w971:T2[])
                n226 = Index Array(array=w971, index=w970) -> (element=w969:T2)
                n227 = Bundle By Name(cluster=w969, "SSL.CACertificateFile"=w967, "SSL.VerifyClient"=TRUE) -> (w968:T2)
                n228 = Replace Array Subset(array=w971, new element=w968, index=w970) -> (w972:T2[])
                n229 = Bundle By Name(cluster=w974, "Servers"=w972) -> (w973:T1)
              }
            }
          }
          frame "SSLCACertificatePath" {
            n230 = Greater Or Equal To 0?(x=w976) -> (x >= 0?=w978:bool)
            n231 = case shown="True" w978 {
              tunnel: w979 -> [_ w982]
              tunnel: w977 -> [w980 w989]
              tunnel: w976 -> [_ w985]
              tunnel: [w980 w988] -> w975
              frame False {
              }
              frame True {
                n232 = Unbundle By Name(w989) -> ("Servers"=w986:T2[])
                n233 = Index Array(array=w986, index=w985) -> (element=w984:T2)
                n234 = Bundle By Name(cluster=w984, "SSL.CACertificatePath"=w982, "SSL.VerifyClient"=TRUE) -> (w983:T2)
                n235 = Replace Array Subset(array=w986, new element=w983, index=w985) -> (w987:T2[])
                n236 = Bundle By Name(cluster=w989, "Servers"=w987) -> (w988:T1)
              }
            }
          }
          frame "NI.ServerName", "ServerName" {
            n237 = Greater Than 0?(x=w991) -> (x > 0?=w990:bool)
            n238 = case shown="True" w990 {
              tunnel: w995 -> [w1000 w1012]
              tunnel: w994 -> [w998 w1013]
              tunnel: w991 -> [w997 w1015]
              tunnel: [w997 w1016] -> w993
              tunnel: [w999 w1010] -> w992
              frame False {
                n239 = Equal To 0?(x=w997) -> (x = 0?=w996:bool)
                n240 = case shown="True" w996 {
                  tunnel: w1000 -> [w1001 w1005]
                  tunnel: [w1001 w1004] -> w999
                  tunnel: w998 -> [_ w1003]
                  tunnel: w997 -> [_ w1002]
                  frame False {
                    # "A second ServerName in a VirtualHost?\nThis case should never happen."
                  }
                  frame True {
                    # "Default Server"
                    n241 = Unbundle By Name(w1005) -> ("Servers"=w1007:T2[])
                    n242 = Index Array(array=w1007, index=w1002) -> (element=w1009:T2)
                    n243 = Bundle By Name(cluster=w1009, "Name"=w1003) -> (w1008:T2)
                    n244 = Replace Array Subset(array=w1007, new element=w1008, index=w1002) -> (w1006:T2[])
                    n245 = Bundle By Name(cluster=w1005, "Servers"=w1006) -> (w1004:T1)
                  }
                }
              }
              frame True {
                # "We are in a VirtualHost"
                n246 = Unbundle By Name(w1012) -> ("Servers"=w1014:T2[])
                n247 = call <vilib>:"FindServerByName.vi"("Servers"=w1014, "Name"=w1013) -> ("Found"=w1018:bool, "Index"=w1017:i32)  [unwired: 12 in]
                n248 = case shown="True" w1018 {
                  tunnel: w1017 -> [_ w1031]
                  tunnel: [w1019 -1 ("CurrentServer")] -> w1016
                  tunnel: w1015 -> [w1019 w1026]
                  tunnel: w1014 -> [w1022 w1032]
                  tunnel: [w1021 w1027] -> w1011
                  tunnel: w1013 -> [w1023 _]
                  frame False {
                    # "It's a new one- just set the name"
                    n249 = Index Array(array=w1022, index=w1019) -> (element=w1024:T2)
                    n250 = Bundle By Name(cluster=w1024, "Name"=w1023) -> (w1020:T2)
                    n251 = Replace Array Subset(array=w1022, new element=w1020, index=w1019) -> (w1021:T2[])
                  }
                  frame True {
                    # "We found one and deleted it\nAll virtual hosts that share a name\nshould also share all settings.\nAll other server specific directives\nwill be ignored until this virtual\nserver ends."
                    n252 = Index Array(array=w1032, index #1=w1031, index #2=w1026) -> (element #1=w1035:T2, element #2=w1029:T2)
                    n253 = Unbundle By Name(w1029) -> ("Interfaces"=w1030:T7[])
                    n254 = Unbundle By Name(w1035) -> ("Interfaces"=w1036:T7[])
                    n255 = Build Array (concatenate)(w1036, w1030) -> (w1034:T7[])
                    n256 = Bundle By Name(cluster=w1035, "Interfaces"=w1034) -> (w1033:T2)
                    n257 = Replace Array Subset(array=w1032, new element=w1033, index=w1031) -> (w1028:T2[])
                    n258 = Delete From Array(array=w1028, index=w1026) -> (array with subset deleted=w1027:T2[])  [unwired: 1 in, 1 out]
                  }
                }
                n259 = Bundle By Name(cluster=w1012, "Servers"=w1011) -> (w1010:T1)
              }
            }
          }
          frame "ServerRoot" {
            n260 = Equal To 0?(x=w1037) -> (x = 0?=w1038:bool)
            n261 = case shown="True" w1038 {
              tunnel: w1041 -> [w1042 w1045]
              tunnel: w1040 -> [_ w1044]
              tunnel: [w1042 w1043] -> w1039
              frame False {
              }
              frame True {
                n262 = Bundle By Name(cluster=w1045, "Root"=w1044) -> (w1043:T1)
              }
            }
          }
          frame "SessionAutoCreate" {
            n263 = Greater Or Equal To 0?(x=w1046) -> (x >= 0?=w1047:bool)
            n264 = case shown="True" w1047 {
              tunnel: w1050 -> [w1051 w1061]
              tunnel: [w1051 w1059] -> w1049
              tunnel: w1048 -> [_ w1054]
              tunnel: w1046 -> [_ w1055]
              frame False {
              }
              frame True {
                n265 = Unbundle By Name(w1061) -> ("Servers"=w1056:T2[])
                n266 = Equal?(x=w1054, y="on") -> (x = y?=w1053:bool)
                n267 = Index Array(array=w1056, index=w1055) -> (element=w1058:T2)
                n268 = Bundle By Name(cluster=w1058, "SessionAutoCreate"=w1053) -> (w1057:T2)
                n269 = Replace Array Subset(array=w1056, new element=w1057, index=w1055) -> (w1060:T2[])
                n270 = Bundle By Name(cluster=w1061, "Servers"=w1060) -> (w1059:T1)
              }
            }
          }
          frame "LimitWorkers", "ThreadLimit", "WorkerLimit" {
            n271 = Equal To 0?(x=w1062) -> (x = 0?=w1063:bool)
            n272 = case shown="True" w1063 {
              tunnel: w1066 -> [w1067 w1071]
              tunnel: [w1067 w1070] -> w1065
              tunnel: w1064 -> [_ w1069]
              frame False {
              }
              frame True {
                n273 = Decimal String To Number(string=w1069) -> (number=w1068:i32)  [unwired: 2 in, 1 out]
                n274 = Bundle By Name(cluster=w1071, "ThreadLimit"=w1068) -> (w1070:T1)
              }
            }
          }
          frame "LimitRequestBody" {
            n275 = Equal To 0?(x=w1072) -> (x = 0?=w1073:bool)
            n276 = case shown="True" w1073 {
              tunnel: w1076 -> [w1077 w1081]
              tunnel: [w1077 w1080] -> w1075
              tunnel: w1074 -> [_ w1079]
              frame False {
              }
              frame True {
                n277 = Decimal String To Number(string=w1079) -> (number=w1078:i32)  [unwired: 2 in, 1 out]
                n278 = Bundle By Name(cluster=w1081, "LimitRequestBody"=w1078) -> (w1080:T1)
              }
            }
          }
          frame "LimitResponseBody" {
            n279 = Equal To 0?(x=w1082) -> (x = 0?=w1083:bool)
            n280 = case shown="True" w1083 {
              tunnel: w1086 -> [w1087 w1091]
              tunnel: [w1087 w1090] -> w1085
              tunnel: w1084 -> [_ w1089]
              frame False {
              }
              frame True {
                n281 = Decimal String To Number(string=w1089) -> (number=w1088:i32)  [unwired: 2 in, 1 out]
                n282 = Bundle By Name(cluster=w1091, "LimitResponseBody"=w1088) -> (w1090:T1)
              }
            }
          }
          frame "InactivityTimeout", "Timeout" {
            n283 = Greater Or Equal To 0?(x=w1092) -> (x >= 0?=w1093:bool)
            n284 = case shown="True" w1093 {
              tunnel: w1096 -> [w1097 w1106]
              tunnel: [w1097 w1104] -> w1095
              tunnel: w1094 -> [_ w1099]
              tunnel: w1092 -> [_ w1100]
              frame False {
              }
              frame True {
                n285 = Unbundle By Name(w1106) -> ("Servers"=w1101:T2[])
                n286 = Decimal String To Number(string=w1099) -> (number=w1098:i32)  [unwired: 2 in, 1 out]
                n287 = Index Array(array=w1101, index=w1100) -> (element=w1103:T2)
                n288 = Bundle By Name(cluster=w1103, "Timeout"=w1098) -> (w1102:T2)
                n289 = Replace Array Subset(array=w1101, new element=w1102, index=w1100) -> (w1105:T2[])
                n290 = Bundle By Name(cluster=w1106, "Servers"=w1105) -> (w1104:T1)
              }
            }
          }
          frame "TypesConfig" {
            n291 = Equal To 0?(x=w1107) -> (x = 0?=w1108:bool)
            n292 = case shown="True" w1108 {
              tunnel: w1111 -> [w1112 w1115]
              tunnel: w1110 -> [_ w1114]
              tunnel: [w1112 w1113] -> w1109
              frame False {
              }
              frame True {
                n293 = Bundle By Name(cluster=w1115, "TypesConfig"=w1114) -> (w1113:T1)
              }
            }
          }
          frame "User" {
            n294 = Equal To 0?(x=w1116) -> (x = 0?=w1117:bool)
            n295 = case shown="True" w1117 {
              tunnel: w1120 -> [w1121 w1124]
              tunnel: w1119 -> [_ w1123]
              tunnel: [w1121 w1122] -> w1118
              frame False {
              }
              frame True {
                n296 = Bundle By Name(cluster=w1124, "User"=w1123) -> (w1122:T1)
              }
            }
          }
          frame "AddOutputFilter", "SetConnector" {
            # "Ignore these directives, as they will always be added at the beginning and end of the pipeline."
          }
          frame Default {
            # "Store any unknown tokens in the current container's\nKey/Value array"
            n297 = Greater Or Equal To 0?(x=w1133) -> (x >= 0?=w1132:bool)
            n298 = Match Pattern(string=w1128, regular expression="\\s*[^#]") -> (offset past match=w1130:i32)  [unwired: 1 in, 3 out]
            n299 = Greater Or Equal To 0?(x=w1130) -> (x >= 0?=w1129:bool)
            n300 = And(x=w1129, y=w1132) -> (x .and. y?=w1131:bool)
            n301 = case shown="True" w1131 {
              tunnel: w1128 -> [_ w1149]
              tunnel: w1136 -> [_ w1148]
              tunnel: w1135 -> [w1137 w1141]
              tunnel: [w1137 w1140] -> w1134
              tunnel: w1133 -> [_ w1139]
              tunnel: w1133 -> [_ w1138]
              frame False {
              }
              frame True {
                n302 = Unbundle By Name(w1141) -> ("Servers"=w1144:T2[])
                n303 = Index Array(array=w1144, index=w1139) -> (element=w1146:T2)
                n304 = Unbundle By Name(w1146) -> ("Key/Value"=w1150:string[][])
                n305 = Build Array(w1149, w1148) -> (w1147:string[])
                n306 = Build Array (concatenate)(w1150, w1147) -> (w1145:string[][])
                n307 = Bundle By Name(cluster=w1146, "Key/Value"=w1145) -> (w1143:T2)
                n308 = Replace Array Subset(array=w1144, new element=w1143, index=w1138) -> (w1142:T2[])
                n309 = Bundle By Name(cluster=w1141, "Servers"=w1142) -> (w1140:T1)
              }
            }
          }
        }
        n310 = Increment(x=w14) -> (x+1=w12:i32)
        n311 = case shown="Error" w13 {
          selector: w13 -> [w26 w27]
          tunnel: [w26 w33] -> w16
          tunnel: "\nError parsing web server configuration file.\nError on line " ("string") -> [_ w30]
          tunnel: w12 -> [_ w29]
          frame No Error {
          }
          frame Error {
            n312 = Unbundle By Name(w27) -> ("source"=w32:string)
            n313 = Number To Decimal String(number=w29) -> (decimal integer string=w28:string)  [unwired: 1 in]
            n314 = Concatenate Strings(w32, w30, w28) -> (w31:string)
            n315 = Bundle By Name(cluster=w27, "source"=w31) -> (w33:errorcluster)
          }
        }
      }
      n316 = Merge Errors(w7) -> (w6:errorcluster)
    }
    frame Error {
    }
  }
  "Config" <- w5
  "error out" <- w2
